vi "2-ReadAllFiles.vi"(8 "error in (no error)":errorcluster, 11 "AllControls IN":T2) -> (0 "error out":errorcluster, 3 "AllControls Out":T2)   [LabVIEW 2017]
uses:
  Ctrls/AllControls.ctl
  Ctrls/TesterInfo.ctl
  <vilib>/Utility/miscctls.llb/LVRowAndColumnTypeDef.ctl
  Ctrls/HD Config.ctl
  Ctrls/Position Config.ctl
  <vilib>/Utility/file.llb/Read Delimited Spreadsheet (string).vi
  ComVIS/Files/Ini/ReadIniFiles_ByVarient.vi
  <vilib>/regexp/Match Regular Expression.xnode
panel:
  in  "TesterInfo":T1
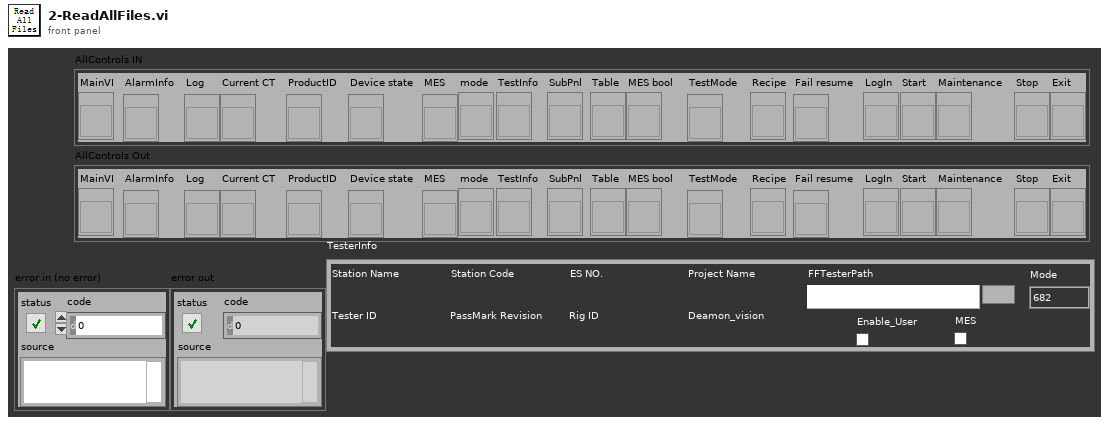
[diagram p1: front panel]
types:
  T1 = typedef "TesterInfo.ctl" = cluster{"Station Name":string, "Station Code":string, "ES NO.":string, "Tester ID":string, "PassMark Revision":string, "Rig ID":string, "Deamon_vision":string, "Project Name":string, "FFTesterPath":path, "Enable_User":bool, "Mode":enum16{"682"}, "MES":bool}
  T2 = typedef "AllControls.ctl" = cluster{"MainVI":refnum<vi>, "AlarmInfo":refnum<vi>, "Log":refnum<vi>, "Current CT":refnum<vi>, "ProductID":refnum<vi>, "Device state":refnum<vi>, "MES":refnum<vi>, "mode":refnum<vi>, "TestInfo":refnum<vi>, "SubPnl":refnum<vi>, "Table":refnum<vi>, "MES bool":refnum<vi>, "TestMode":refnum<vi>, "Recipe":refnum<vi>, "Fail resume":refnum<vi>, "LogIn":refnum<vi>, "Start":refnum<vi>, "Maintenance":refnum<vi>, "Stop":refnum<vi>, "Exit":refnum<vi>}
  T3 = typedef "Position Config.ctl" = cluster{"OrificeSize_12.7":i32, "OrificeSize_13":i32, "OrificeSize_30":i32, "OrificeSize_16":i32}
  T4 = typedef "HD Config.ctl" = cluster{" PC":cluster{"PC Address":u8[], "PC Port":i32}, "FCO":cluster{"COM":refnum<visa-resource-name>, "Baudrate":u32}, "DC Power ":cluster{"COM":refnum<visa-resource-name>, "Baudrate":u32}, "PW3336":cluster{"COM":refnum<visa-resource-name>, "Baudrate":u32}, "Lefoo":cluster{"COM":refnum<visa-resource-name>, "Baudrate":u32}, "AI Model":cluster{"COM":refnum<visa-resource-name>, "Baudrate":u32}, "DIPC":cluster{"COM":refnum<visa-resource-name>}, "RFID":cluster{"IP Address":string, "Port":u16, "Retry":u16}, "Motor":cluster{"COM":refnum<visa-resource-name>, "Baudrate":u32}, "Fail_resume_mode":bool, "GRR":bool}
  T5 = typedef "LVRowAndColumnTypeDef.ctl" = cluster{"Row":i32, "Column":i32}
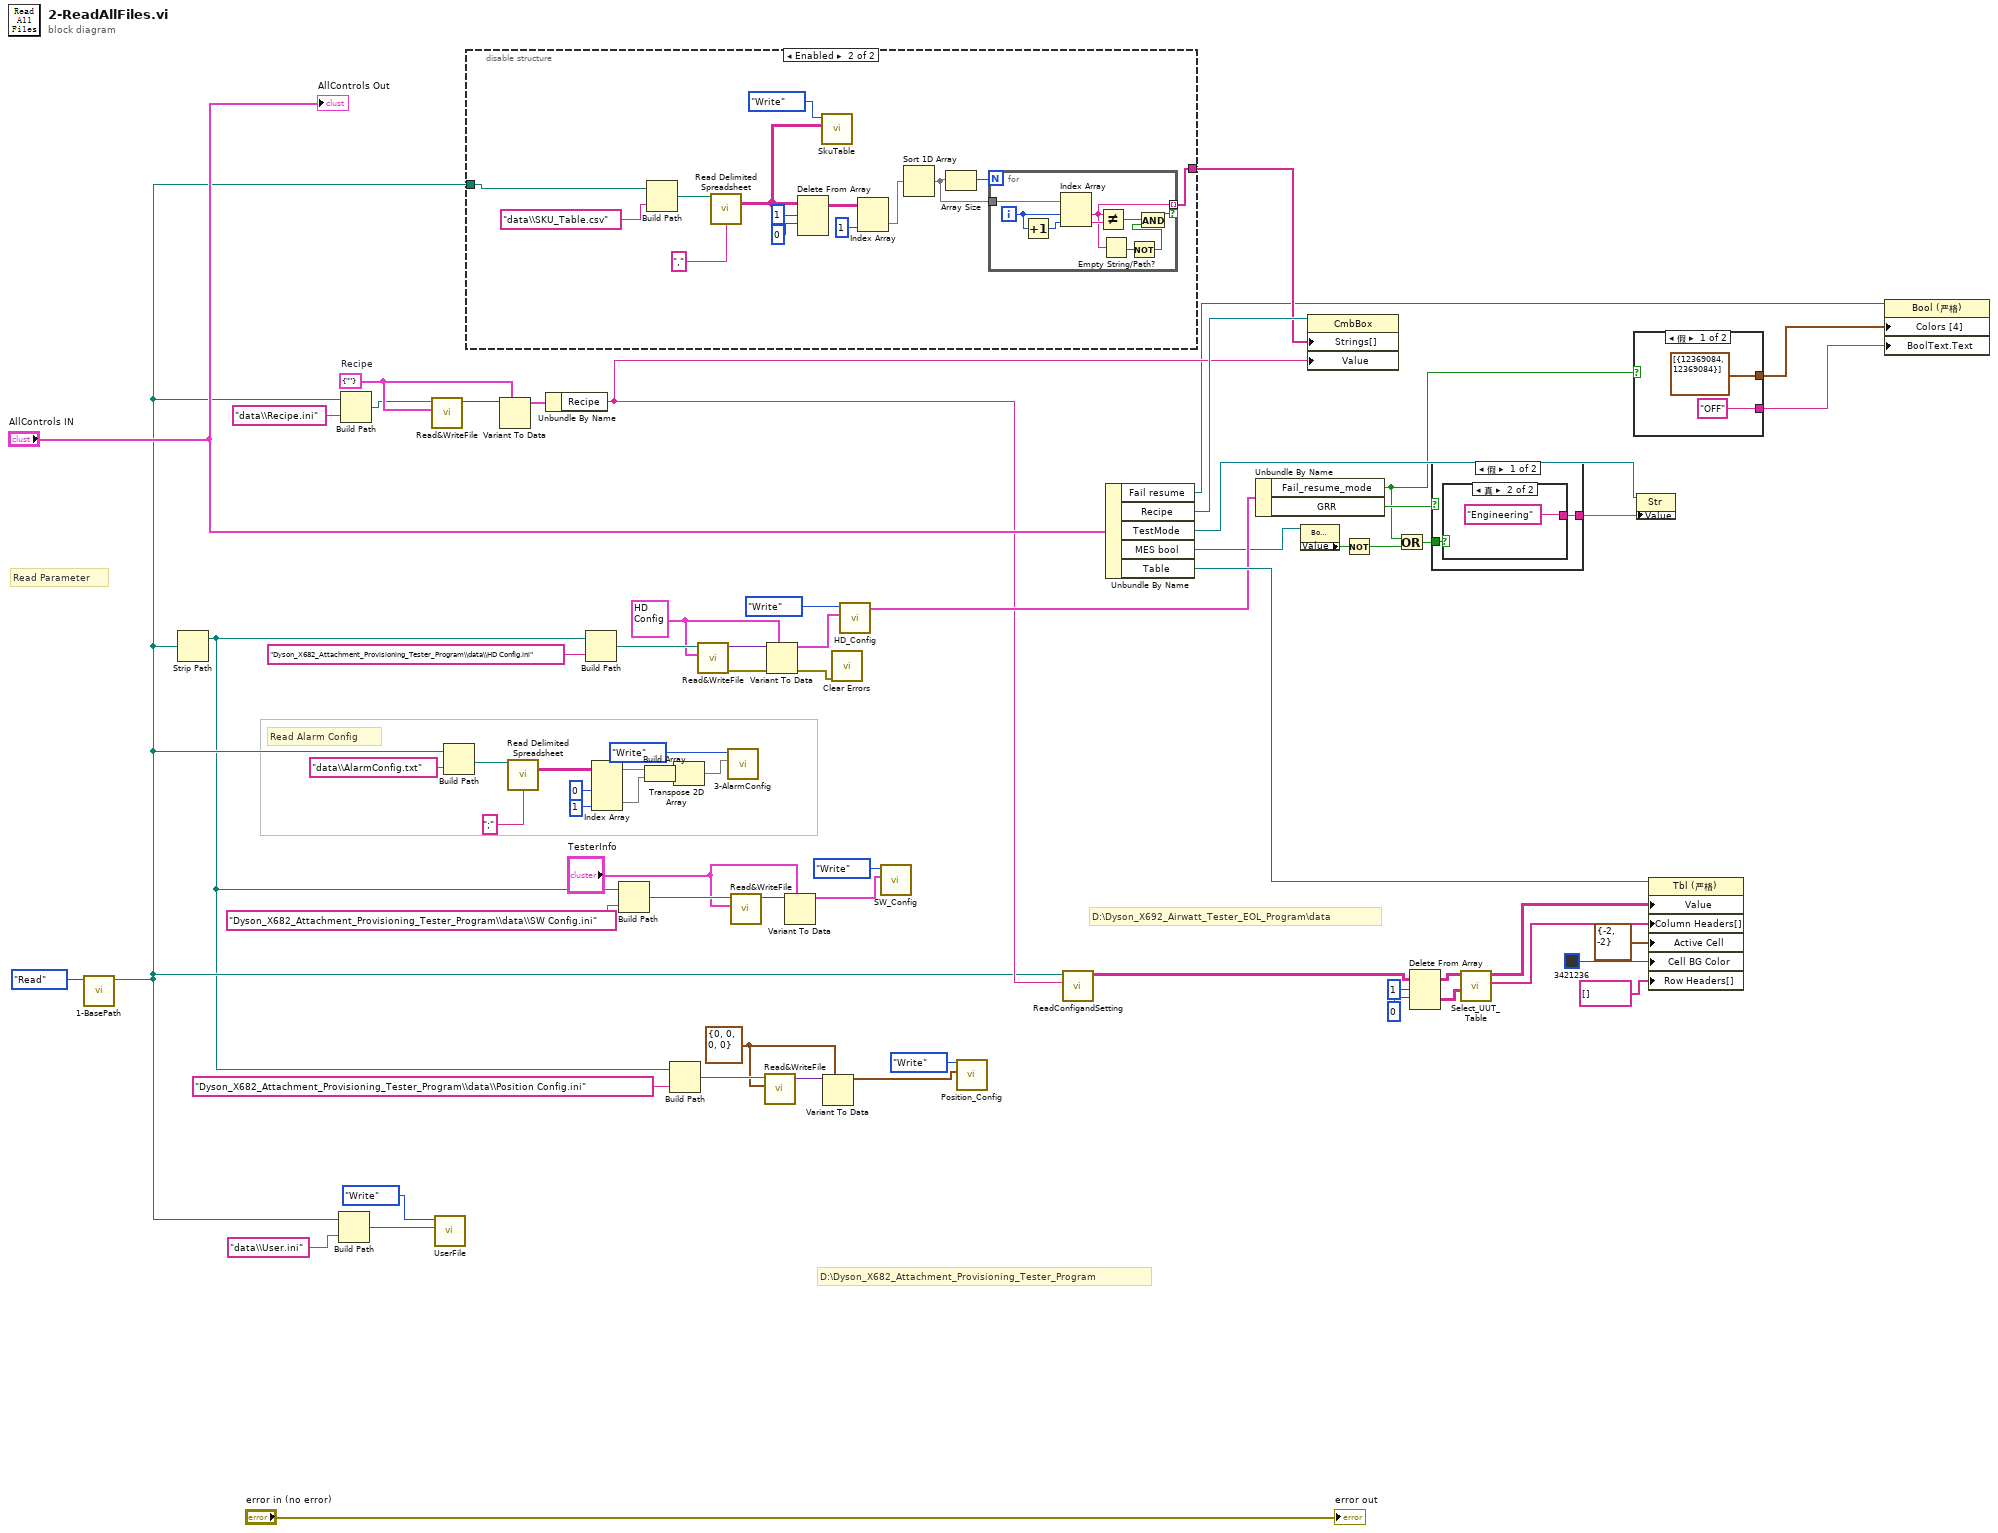
[diagram p0: block diagram]
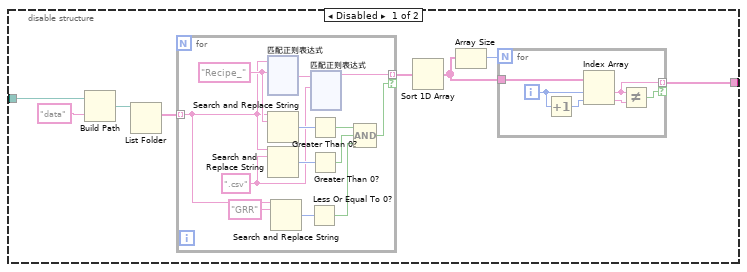
[diagram p2: hidden frame]
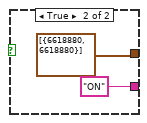
[diagram p3: hidden frame]
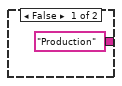
[diagram p4: hidden frame]
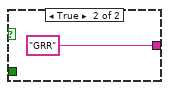
[diagram p5: hidden frame]
diagram:
  w8 = T3 {"OrificeSize_12.7"=0, "OrificeSize_13"=0, "OrificeSize_30"=0, "OrificeSize_16"=0} ("Position Config")
  w24 = cluster{"Recipe":string} {"Recipe"=""}  # Recipe
  w36 = T4 {" PC"={"PC Address"=[], "PC Port"=0}, "FCO"={"COM"="", "Baudrate"=0}, "DC Power "={"COM"="", "Baudrate"=0}, "PW3336"={"COM"="", "Baudrate"=0}, "Lefoo"={"COM"="", "Baudrate"=0}, "AI Model"={"COM"="", "Baudrate"=0}, "DIPC"={"COM"=""}, "RFID"={"IP Address"="", "Port"=0, "Retry"=0}, "Motor"={"COM"="", "Baudrate"=0}, "Fail_resume_mode"=FALSE, "GRR"=FALSE} ("HD Config")
  # "D:\\Dyson_X682_Attachment_Provisioning_Tester_Program"
  # "D:\\Dyson_X692_Airwatt_Tester_EOL_Program\\data"
  # "Read Alarm Config"
  # "Read Parameter"
  n1 = call "1-BasePath.vi"("Step"=enum16{"Initial", "Write", "Read"}."Read") -> ("Path Out"=w14:path)  [unwired: 9 in, 1 out]
  n2 = Strip Path(path=w14) -> (stripped path=w13:path)  [unwired: 1 out]
  n3 = Build Path(base path=w14, name or relative path="data\\User.ini") -> (appended path=w50:path)
  n4 = Build Path(base path=w14, name or relative path="data\\Recipe.ini") -> (appended path=w21:path)
  n5 = call-poly "Read&WriteFile.vi"("Varient"=w24, "path"=w21) -> ("DataOut"=w25:variant)  [unwired: 8 in, 1 out]
  n6 = call "UserFile.vi"("UserPath in"=w50, "Step"=enum16{"Initial", "Write", "Read"}."Write") -> ()  [unwired: 8 in, 2 out]
  n7 = Build Path(base path=w14, name or relative path="data\\AlarmConfig.txt") -> (appended path=w61:path)
  n8 = disable-structure shown="Enabled" {
    disable-tunnel: [w72 w328] -> w26
    disable-tunnel: w14 -> [w71 w335]
    frame Disabled {
      n9 = Build Path(base path=w71, name or relative path="data") -> (appended path=w77:path)
      n10 = List Folder(path=w77) -> (filenames=w76:string[])  [unwired: 3 in, 3 out]
      n11 = for {
        tunnel: w76 -> [w88] mode=indexing
        tunnel: [w89] -> w75 mode=indexing if=w95
        w90 = ".csv" ("搜索字符串")
        w92 = "Recipe_" ("搜索字符串")
        n12 = xnode "匹配正则表达式"("输入字符串"=w88, "正则表达式"=w92) -> ("匹配之后"=w91:string)  [unwired: 4 in, 4 out]
        n13 = Search and Replace String(input string=w88, search string=w92) -> (number of replacements=w97:i32)  [unwired: 6 in, 3 out]
        n14 = Search and Replace String(input string=w88, search string=w90) -> (number of replacements=w94:i32)  [unwired: 6 in, 3 out]
        n15 = Search and Replace String(input string=w88, search string="GRR" ("搜索字符串")) -> (number of replacements=w86:i32)  [unwired: 6 in, 3 out]
        n16 = Less Or Equal To 0?(x=w86) -> (x <= 0?=w85:bool)
        n17 = Greater Than 0?(x=w97) -> (x > 0?=w96:bool)
        n18 = Greater Than 0?(x=w94) -> (x > 0?=w93:bool)
        n19 = xnode "匹配正则表达式"("输入字符串"=w91, "正则表达式"=w90) -> ("匹配之前"=w89:string)  [unwired: 4 in, 4 out]
        n20 = Compound Arithmetic op=AND ("复合运算")(w96, w93, w85) -> (w95:bool)
      }
      n21 = Sort 1D Array(array=w75) -> (sorted array=w73:string[])
      n22 = Array Size(array=w73) -> (size(s)=w74:i32)
      n23 = for {
        N: w74 -> [_]
        tunnel: w73 -> [w84]
        tunnel: [w80] -> w72 mode=indexing if=w83
        i -> [w82]
        n24 = Increment(x=w82) -> (x+1=w81:i32)
        n25 = Index Array(array=w84, index #1=w82, index #2=w81) -> (element #1=w80:string, element #2=w79:string)
        n26 = Not Equal?(x=w80, y=w79) -> (x != y?=w83:bool)
      }
    }
    frame Enabled {
      n27 = Build Path(base path=w335, name or relative path="data\\SKU_Table.csv") -> (appended path=w339:path)
      n28 = call-poly <vilib>:"Read Delimited Spreadsheet.vi"("file path (dialog if empty)"=w339, "delimiter (\\t)"="," ("delimiter (\\t)")) -> ("all rows"=w334:string[][])  [unwired: 8 in, 5 out]
      n29 = Delete From Array(array=w334, length=1 ("长度"), index (row)=0 ("索引 (行)")) -> (array with subset deleted=w331:string[][])  [unwired: 1 in, 1 out]
      n30 = call "SkuTable.vi"("Tabledata in"=w334, "Step"=enum16{"Initial", "Write", "Read"}."Write") -> ()  [unwired: 8 in, 2 out]
      n31 = Index Array(array=w331, index (col)=1 ("禁用的索引 (列)")) -> (element=w326:string[])  [unwired: 1 in]
      n32 = Sort 1D Array(array=w326) -> (sorted array=w327:string[])
      n33 = Array Size(array=w327) -> (size(s)=w329:i32)
      n34 = for {
        N: w329 -> [_]
        tunnel: w327 -> [w348]
        tunnel: [w343] -> w328 mode=indexing if=w341
        i -> [w346]
        n35 = Increment(x=w346) -> (x+1=w345:i32)
        n36 = Index Array(array=w348, index #1=w346, index #2=w345) -> (element #1=w343:string, element #2=w344:string)
        n37 = Not Equal?(x=w343, y=w344) -> (x != y?=w347:bool)
        n38 = Empty String/Path?(string/path=w343) -> (empty?=w342:bool)
        n39 = Not(x=w342) -> (.not. x?=w340:bool)
        n40 = And(x=w347, y=w340) -> (x .and. y?=w341:bool)
      }
    }
  }
  n41 = Variant To Data(type=w24, Variant=w25) -> (data=w23:cluster{"Recipe":string})  [unwired: 1 in, 1 out]
  n42 = call-poly <vilib>:"Read Delimited Spreadsheet.vi"("file path (dialog if empty)"=w61, "delimiter (\\t)"=";" ("delimiter (\\t)")) -> ("all rows"=w58:string[][])  [unwired: 8 in, 5 out]
  n43 = Unbundle By Name(w23) -> ("Recipe"=w20:string)
  n44 = Build Path(base path=w13, name or relative path="Dyson_X682_Attachment_Provisioning_Tester_Program\\data\\HD Config.ini") -> (appended path=w66:path)
  n45 = Index Array(array=w58, index (col) #1=0 ("disabled index (col)"), index (col) #2=1 ("index (col)")) -> (element #1=w57:string[], element #2=w53:string[])  [unwired: 2 in]
  n46 = Build Path(base path=w13, name or relative path="Dyson_X682_Attachment_Provisioning_Tester_Program\\data\\SW Config.ini") -> (appended path=w5:path)
  n47 = Build Array(w57, w53) -> (w54:string[][])
  n48 = Build Path(base path=w13, name or relative path="Dyson_X682_Attachment_Provisioning_Tester_Program\\data\\Position Config.ini") -> (appended path=w11:path)
  n49 = Transpose 2D Array(2D array=w54) -> (transposed array=w52:string[][])
  n50 = call-poly "Read&WriteFile.vi"("Varient"=w36, "path"=w66) -> ("error out"=w64:errorcluster, "DataOut"=w65:variant)  [unwired: 8 in]
  n51 = call "3-AlarmConfig.vi"("AlarmConfig In"=w52, "Step"=enum16{"Initial", "Write", "Read"}."Write") -> ()  [unwired: 8 in, 2 out]
  n52 = call-poly "Read&WriteFile.vi"("Varient"="TesterInfo", "path"=w5) -> ("DataOut"=w3:variant)  [unwired: 8 in, 1 out]
  n53 = call-poly "Read&WriteFile.vi"("Varient"=w8, "path"=w11) -> ("DataOut"=w9:variant)  [unwired: 8 in, 1 out]
  n54 = Variant To Data(error in=w64, type=w36, Variant=w65) -> (data=w48:T4, error out=w63:errorcluster)
  n55 = Variant To Data(type="TesterInfo", Variant=w3) -> (data=w2:T1)  [unwired: 1 in, 1 out]
  n56 = Variant To Data(type=w8, Variant=w9) -> (data=w7:T3)  [unwired: 1 in, 1 out]
  n57 = call <vilib>:"Clear Errors.vi"("error in (no error)"=w63) -> ()  [unwired: 5 in, 2 out]
  n58 = call "HD_Config.vi"("HD Config in"=w48, "Step"=enum16{"Initial", "Write", "Read"}."Write") -> ("HD Config out"=w35:T4)  [unwired: 8 in, 1 out]
  n59 = call "SW_Config.vi"("SW Config In"=w2, "Step"=enum16{"Initial", "Write", "Read"}."Write") -> ()  [unwired: 8 in, 2 out]
  n60 = call "Position_Config.vi"("Position Config"=w7, "Step"=enum16{"Initial", "Write", "Read"}."Write") -> ()  [unwired: 8 in, 2 out]
  n61 = call "ReadConfigandSetting.vi"("Recipe"=w20, "Path Out"=w14) -> ("TableData"=w40:string[][])  [unwired: 7 in, 2 out]
  n62 = Unbundle By Name("AllControls IN") -> ("Fail resume"=w17:refnum<vi>, "Recipe"=w27:refnum<vi>, "TestMode"=w32:refnum<vi>, "MES bool"=w33:refnum<vi>, "Table"=w42:refnum<vi>)
  n63 = Unbundle By Name(w35) -> ("Fail_resume_mode"=w18:bool, "GRR"=w34:bool)
  n64 = property class="Bool (严格)"(reference=w33) -> ("Value"=w30:bool)  [unwired: 1 in, 2 out]
  n65 = property class="CmbBox"(reference=w27, "Strings[]"=w26, "Value"=w20) -> ()  [unwired: 1 in, 2 out]
  n66 = Not(x=w30) -> (.not. x?=w28:bool)
  n67 = Or(x=w18, y=w28) -> (x .or. y?=w29:bool)
  n68 = Delete From Array(array=w40, length=1 ("长度"), index (row)=0 ("索引 (行)")) -> (deleted portion=w38:string[][], array with subset deleted=w41:string[][])  [unwired: 1 in]
  n69 = case shown="假" w34 {
    tunnel: w29 -> [w350 _]
    tunnel: [w349 "GRR"] -> w31
    frame False {
      n70 = case shown="真" w350 {
        tunnel: ["Production" "Engineering"] -> w349
        frame False {
        }
        frame True {
        }
      }
    }
    frame True {
    }
  }
  n71 = call "Select_UUT_Table.vi"("all Title"=w38, "all Table"=w41) -> ("Title"=w39:string[], "Table"=w19:string[][])  [unwired: 8 in]
  n72 = case shown="假" w18 {
    tunnel: [cluster{u32, u32}[] [{12369084, 12369084}] cluster{u32, u32}[] [{6618880, 6618880}]] -> w16
    tunnel: ["OFF" "ON"] -> w15
    frame False {
    }
    frame True {
    }
  }
  n73 = property class="Str"(reference=w32, "Value"=w31) -> ()  [unwired: 1 in, 2 out]
  n74 = property class="Tbl (严格)"(reference=w42, "Value"=w19, "Column Headers[]"=w39, "Active Cell"=T5 {"Row"=-2, "Column"=-2} ("活动单元格:活动单元格"), "Cell BG Color"=u32 3421236, "Row Headers[]"=string[] [] ("Row Header Strings[]")) -> ()  [unwired: 1 in, 2 out]
  n75 = property on="属性节点" class="Bool (严格)"(reference=w17, "Colors [4]"=w16, "BoolText.Text"=w15) -> ()  [unwired: 1 in, 2 out]
  "AllControls Out" <- "AllControls IN"
  "error out" <- "error in (no error)"
